vi "LVFunction_Imop_GetSoftwareConfig.vi"(0 "WFS_setupfile_IN":path, 11 "error in":errorcluster) -> (4 "WFS_setupfile_OUT":path, 6 "SoftwareOptions":T1, 15 "error out":errorcluster)   [LabVIEW 2020]
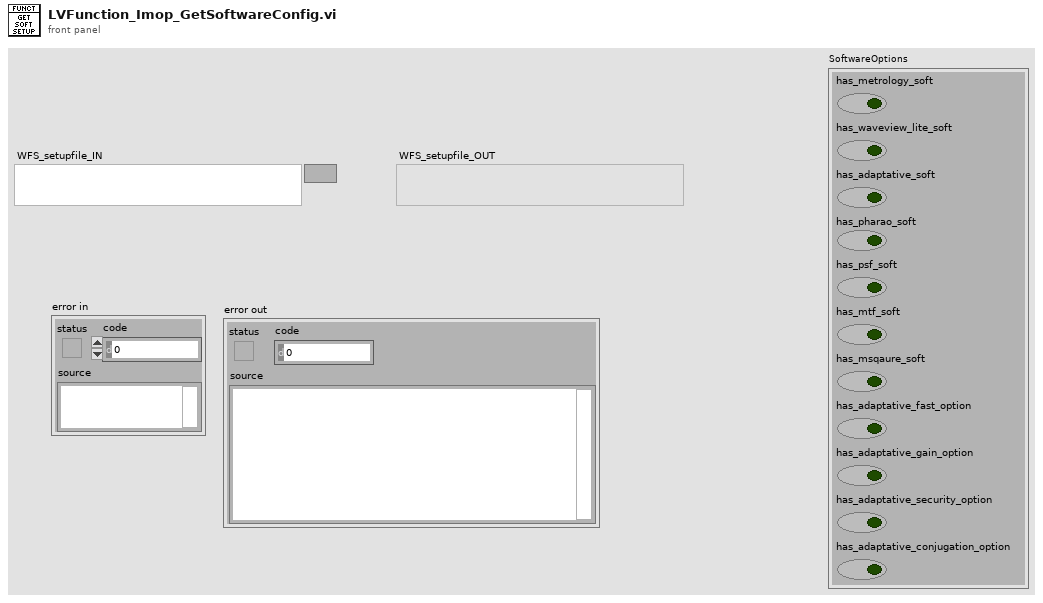
[diagram p1: front panel]
types:
  T1 = cluster{"has_metrology_soft":bool, "has_waveview_lite_soft":bool, "has_adaptative_soft":bool, "has_pharao_soft":bool, "has_psf_soft":bool, "has_mtf_soft":bool, "has_msqaure_soft":bool, "has_adaptative_fast_option":bool, "has_adaptative_gain_option":bool, "has_adaptative_security_option":bool, "has_adaptative_conjugation_option":bool}
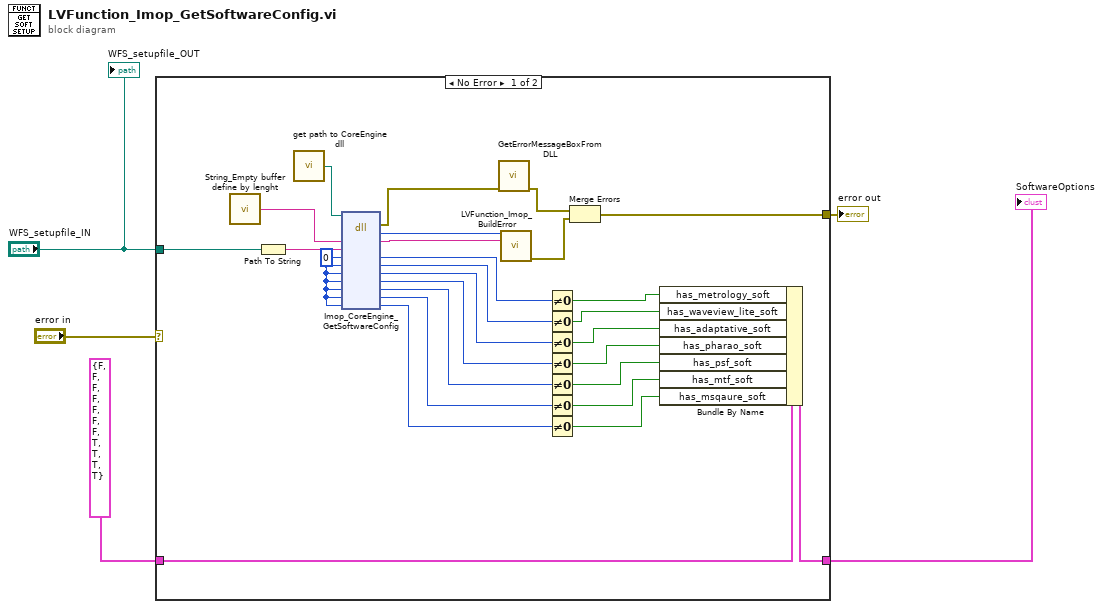
[diagram p0: block diagram]
diagram:
  n1 = case shown="No Error" "error in" {
    selector: "error in" -> [_ w34]
    tunnel: [w25 w34] -> w4
    tunnel: "WFS_setupfile_IN" -> [w24 _]
    tunnel: T1 {"has_metrology_soft"=FALSE, "has_waveview_lite_soft"=FALSE, "has_adaptative_soft"=FALSE, "has_pharao_soft"=FALSE, "has_psf_soft"=FALSE, "has_mtf_soft"=FALSE, "has_msqaure_soft"=FALSE, "has_adaptative_fast_option"=TRUE, "has_adaptative_gain_option"=TRUE, "has_adaptative_security_option"=TRUE, "has_adaptative_conjugation_option"=TRUE} ("SoftwareOptions") -> [w15 w33]
    tunnel: [w14 w33] -> w2
    frame No Error {
      w6 = u8 0 ("has_metrology_soft")
      n2 = call "String_Empty buffer define by lenght.vi"() -> ("Empty buffer"=w26:string)  [unwired: 1 in]
      n3 = Path To String(path=w24) -> (string=w23:string)
      n4 = call "get path to CoreEngine dll.vi"() -> ("path to wavekit library"=w29:path)  [unwired: 14 in, 1 out]
      n5 = dll-call lib="D:/soft/HASO_v3/SVN_trunk/ImOpCoreEngine4_LV2011/DLLs/c_interface_vc100.dll" fn="Imop_CoreEngine_GetSoftwareConfig"(path in=w29, "message"=w26, "config_file_path"=w23, "has_metrology_soft"=w6, "has_waveview_lite_soft"=w6, "has_adaptative_soft"=w6, "has_pharao_soft"=w6, "has_psf_soft"=w6, "has_mtf_soft"=w6, "has_msquare_soft"=w6) -> (error out=w30:errorcluster, "return type"=w28:i32, "message"=w27:string, "has_metrology_soft"=w22:u8, "has_waveview_lite_soft"=w17:u8, "has_adaptative_soft"=w20:u8, "has_pharao_soft"=w16:u8, "has_psf_soft"=w21:u8, "has_mtf_soft"=w19:u8, "has_msquare_soft"=w18:u8)  [unwired: 3 in, 1 out]
      n6 = call "GetErrorMessageBoxFromDLL.vi"("error IN"=w30) -> ("error OUT"=w31:errorcluster)  [unwired: 10 in]
      n7 = call "LVFunction_Imop_BuildError.vi"("code"=w28, "String to Prepend to source (\"\")"=w27) -> ("error out"=w32:errorcluster)  [unwired: 13 in]
      n8 = Not Equal To 0?(x=w22) -> (x != 0?=w13:bool)
      n9 = Not Equal To 0?(x=w17) -> (x != 0?=w12:bool)
      n10 = Not Equal To 0?(x=w20) -> (x != 0?=w11:bool)
      n11 = Not Equal To 0?(x=w16) -> (x != 0?=w10:bool)
      n12 = Not Equal To 0?(x=w21) -> (x != 0?=w9:bool)
      n13 = Not Equal To 0?(x=w19) -> (x != 0?=w8:bool)
      n14 = Not Equal To 0?(x=w18) -> (x != 0?=w7:bool)
      n15 = Merge Errors(w31, w32) -> (w25:errorcluster)
      n16 = Bundle By Name(cluster=w15, "has_metrology_soft"=w13, "has_waveview_lite_soft"=w12, "has_adaptative_soft"=w11, "has_pharao_soft"=w10, "has_psf_soft"=w9, "has_mtf_soft"=w8, "has_msqaure_soft"=w7) -> (w14:T1)
    }
    frame Error {
    }
  }
  "error out" <- w4
  "SoftwareOptions" <- w2
  "WFS_setupfile_OUT" <- "WFS_setupfile_IN"
